vi "FGV-Core.vi"(6 "Enum":T1, 8 "error in (no error)":errorcluster, 10 "csm":string, 11 "VI in":refnum<vi>) -> (0 "error out":errorcluster, 2 "Variant":variant, 3 "Path":path)   [LabVIEW 2020, in "CSM-ModuleManager.lvlib"]
uses:
  CSM-ModuleManager.lvlib
  <userlib>/_NEVSTOP/Communicable State Machine(CSM)/addons/INI-Static-Variable-Support/INI-Static-Variable-Support.lvlib
  <userlib>/_NEVSTOP/Communicable State Machine(CSM)/addons/Logger/CSM File Logger.lvlib
  Operation.ctl
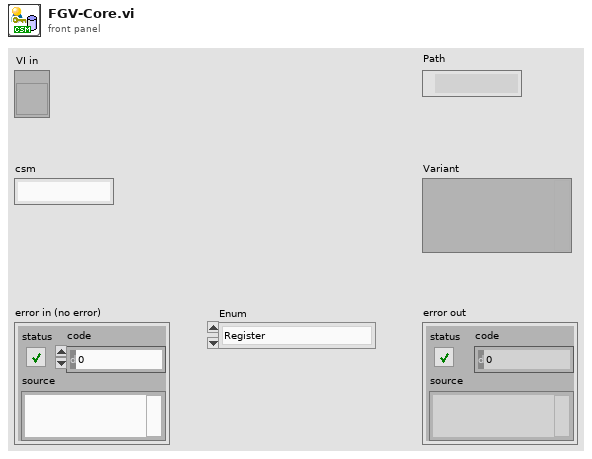
[diagram p1: front panel]
types:
  T1 = typedef "CSM-ModuleManager.lvlib/Operation.ctl" = enum16{"Register", "UnRegister", "Load Config", "Get"}
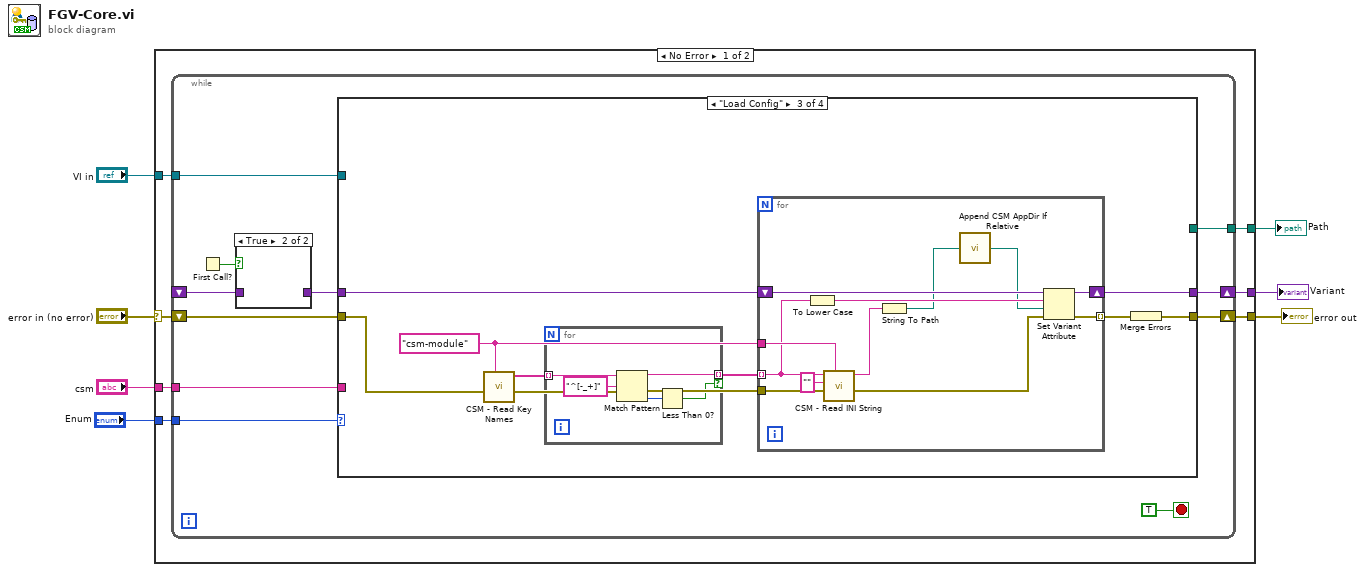
[diagram p0: block diagram]
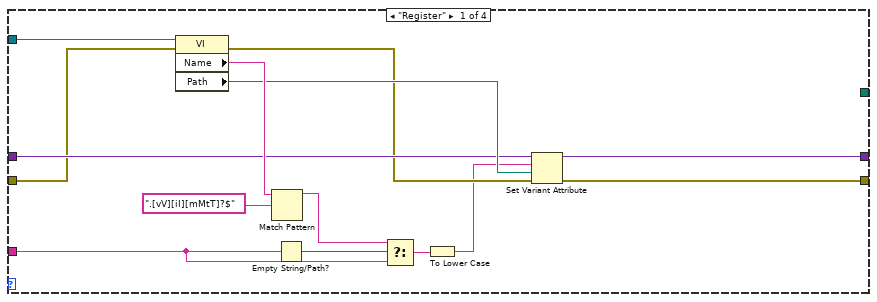
[diagram p3: hidden frame]
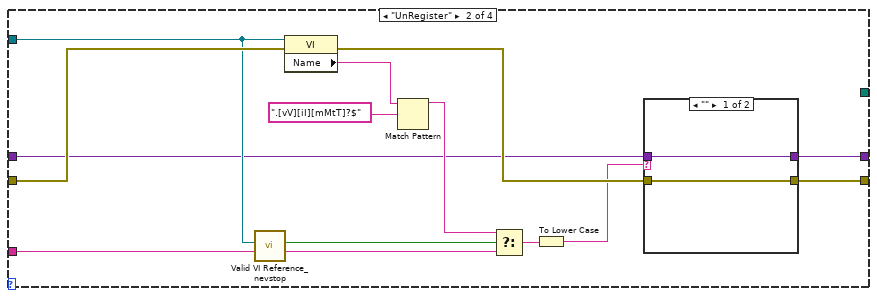
[diagram p4: hidden frame]
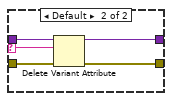
[diagram p5: hidden frame]
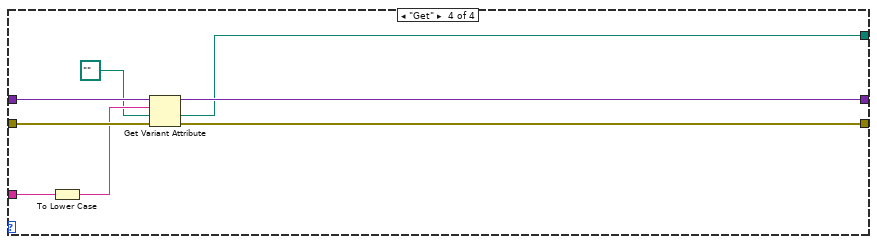
[diagram p6: hidden frame]
diagram:
  n1 = case shown="No Error" "error in (no error)" {
    selector: "error in (no error)" -> [w11 w95]
    tunnel: [w14 w95] -> w7
    tunnel: "csm" -> [w13 _]
    tunnel: "VI in" -> [w12 _]
    tunnel: "Enum" -> [w10 _]
    tunnel: [w9 _] -> w2
    tunnel: [w8 _] -> w1
    frame No Error {
      n2 = while {
        tunnel: w13 -> [w23]
        tunnel: w12 -> [w22]
        shift-right: [w24] -> w8
        shift-left: _ -> [w17]
        shift-right: [w25] -> w14
        shift-left: w11 -> [w21]
        tunnel: w10 -> [w19]
        tunnel: [w15] -> w9
        stop <- TRUE stop-if-true
        n3 = First Call?() -> (First Call?: T/F=w18:bool)
        n4 = case shown="True" w18 {
          tunnel: w17 -> [w26 _]
          tunnel: [w26 _] -> w16
          frame False {
          }
          frame True {
          }
        }
        n5 = case shown="\"Load Config\"" w19 {
          tunnel: [w40 w53 w61 w91] -> w25
          tunnel: [w39 w52 w65 w93] -> w24
          tunnel: w23 -> [w36 w49 _ w90]
          tunnel: w22 -> [w33 w44 _ _]
          tunnel: w16 -> [w32 w43 w64 w94]
          tunnel: w21 -> [w31 w48 w63 w92]
          tunnel: [_ _ _ w87] -> w15
          frame "Register" {
            n6 = property on="Property Node" class="VI"(reference=w33, error in=w31) -> (error out=w30:errorcluster, "Name"=w37:string, "Path"=w34:path)  [unwired: 1 out]
            n7 = Match Pattern(string=w37, regular expression=".[vV][iI][mMtT]?$") -> (before substring=w29:string)  [unwired: 1 in, 3 out]
            n8 = Empty String/Path?(string/path=w36) -> (empty?=w35:bool)
            n9 = Select(t=w29, s=w35, f=w36) -> (s? t:f=w38:string)
            n10 = To Lower Case(string=w38) -> (all lower case string=w27:string)
            n11 = Set Variant Attribute(Variant=w32, name=w27, value=w34, error in=w30) -> (Variant out=w39:variant, error out=w40:errorcluster)  [unwired: 1 out]
          }
          frame "UnRegister" {
            n12 = call <userlib>:"Valid VI Reference_nevstop.vi"("VI Refnum"=w44) -> ("Valid?"=w42:bool)  [unwired: 9 in]
            n13 = property on="Property Node" class="VI"(reference=w44, error in=w48) -> (error out=w47:errorcluster, "Name"=w50:string)  [unwired: 1 out]
            n14 = Match Pattern(string=w50, regular expression=".[vV][iI][mMtT]?$") -> (before substring=w46:string)  [unwired: 1 in, 3 out]
            n15 = Select(t=w46, s=w42, f=w49) -> (s? t:f=w51:string)
            n16 = To Lower Case(string=w51) -> (all lower case string=w41:string)
            n17 = case shown="\"\"" w41 {
              selector: w41 -> [_ w56]
              tunnel: [w54 w60] -> w53
              tunnel: [w55 w59] -> w52
              tunnel: w47 -> [w54 w58]
              tunnel: w43 -> [w55 w57]
              frame "" {
              }
              frame Default {
                n18 = Delete Variant Attribute(4:w58, 6:w56, 7:w57) -> (0:w60:errorcluster, 3:w59:variant)  [unwired: 1 out]
              }
            }
          }
          frame "Load Config" {
            w68 = "csm-module" ("Section Name (\"\" as Default)")
            n19 = call <userlib>:"CSM - Read Key Names.vi"("Section Name (\"\" as Default)"=w68, "error in (no error)"=w63) -> ("error out"=w69:errorcluster, "Keys"=w66:string[])  [unwired: 6 in]
            n20 = for {
              tunnel: [w85] -> w67 mode=indexing if=w82
              tunnel: w66 -> [w86] mode=indexing
              n21 = Match Pattern(string=w86, regular expression="^[-_+]") -> (before substring=w85:string, offset past match=w83:i32)  [unwired: 1 in, 2 out]
              n22 = Less Than 0?(x=w83) -> (x < 0?=w82:bool)
            }
            n23 = for {
              tunnel: w69 -> [w81]
              tunnel: w68 -> [w80]
              tunnel: w67 -> [w74] mode=indexing
              shift-right: [w78] -> w65
              shift-left: w64 -> [w79]
              tunnel: [w75] -> w62 mode=indexing
              n24 = To Lower Case(string=w74) -> (all lower case string=w73:string)
              n25 = call <userlib>:"CSM - Read INI String.vi"("Section Name (\"\" as Default)"=w80, "error in (no error)"=w81, "Default Value"="", "Variable Name"=w74) -> ("error out"=w76:errorcluster, "Value"=w72:string)  [unwired: 3 in, 1 out]
              n26 = String To Path(string=w72) -> (path=w71:path)
              n27 = call <userlib>:"Append CSM AppDir If Relative.vi"("Relative Path (.)"=w71) -> ("Application Directory (+ Relative)"=w70:path)  [unwired: 4 in]
              n28 = Set Variant Attribute(Variant=w79, name=w73, value=w70, error in=w76) -> (Variant out=w78:variant, error out=w75:errorcluster)  [unwired: 1 out]
            }
            n29 = Merge Errors(w62) -> (w61:errorcluster)
          }
          frame "Get" {
            n30 = To Lower Case(string=w90) -> (all lower case string=w89:string)
            n31 = Get Variant Attribute(Variant=w94, name=w89, default value (empty Variant)=path "", error in=w92) -> (duplicate Variant=w93:variant, value=w87:path, error out=w91:errorcluster)  [unwired: 1 out]
          }
        }
      }
    }
    frame Error {
    }
  }
  "error out" <- w7
  "Path" <- w2
  "Variant" <- w1
